vi "load_automatic.vi"(8 "error in (no error)":errorcluster) -> (0 "error out":errorcluster, 2 "replaced_step(s)":bool, 3 "automatic_steps out":variant)   [LabVIEW 2015, in "example_01.lvlib"]
doc: "load_automatic.vi will add automatic steps as variant attributes to an empty variant."
uses:
  example_01.lvlib
  <userlib>/antonio-alexander/lv-recipe-machine/public/_controls/step.ctl
  <userlib>/antonio-alexander/lv-recipe-machine/public/_controls/vi_reference_type.ctl
  _controls/steps_actions.ctl
  <userlib>/antonio-alexander/lv-recipe-machine/public/_controls/vi_reference_automatic_step.ctl
  <userlib>/antonio-alexander/lv-recipe-machine/public/_controls/vi_reference_criteria.ctl
  <userlib>/antonio-alexander/lv-recipe-machine/public/_controls/vi_reference_launch.ctl
  <userlib>/antonio-alexander/lv-recipe-machine/public/_controls/vi_reference_manual_action.ctl
  <userlib>/antonio-alexander/lv-recipe-machine/public/_controls/vi_reference_transition.ctl
  <userlib>/antonio-alexander/lv-recipe-machine/lv-recipe-machine.lvlib
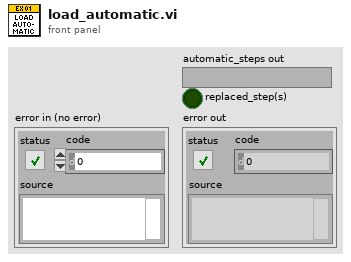
[diagram p1: front panel]
types:
  T1 = typedef "lv-recipe-machine.lvlib/vi_reference_type.ctl" = enum16{"<vi_reference_type>", "manual_action", "auto_step", "auto_criteria", "auto_transition", "auto_launcher", "<null>"}
  T2 = typedef "lv-recipe-machine.lvlib/vi_reference_transition.ctl" = refnum<vi>
  T3 = typedef "lv-recipe-machine.lvlib/vi_reference_manual_action.ctl" = refnum<vi>
  T4 = typedef "lv-recipe-machine.lvlib/vi_reference_launch.ctl" = refnum<vi>
  T5 = typedef "lv-recipe-machine.lvlib/vi_reference_criteria.ctl" = refnum<vi>
  T6 = typedef "lv-recipe-machine.lvlib/vi_reference_automatic_step.ctl" = refnum<vi>
  T7 = typedef "example_01.lvlib/steps_actions.ctl" = enum16{"<steps_actions>", "manual_random", "manual_comparison", "manual_wait", "auto_random", "auto_wait", "criteria_initialize", "criteria_count", "criteria_comparison", "transition_simple", "transition_count", "transition_comparison", "launch_wait", "<null>"}
  T8 = typedef "lv-recipe-machine.lvlib/step.ctl" = cluster{"name":string, "vi_reference":variant}
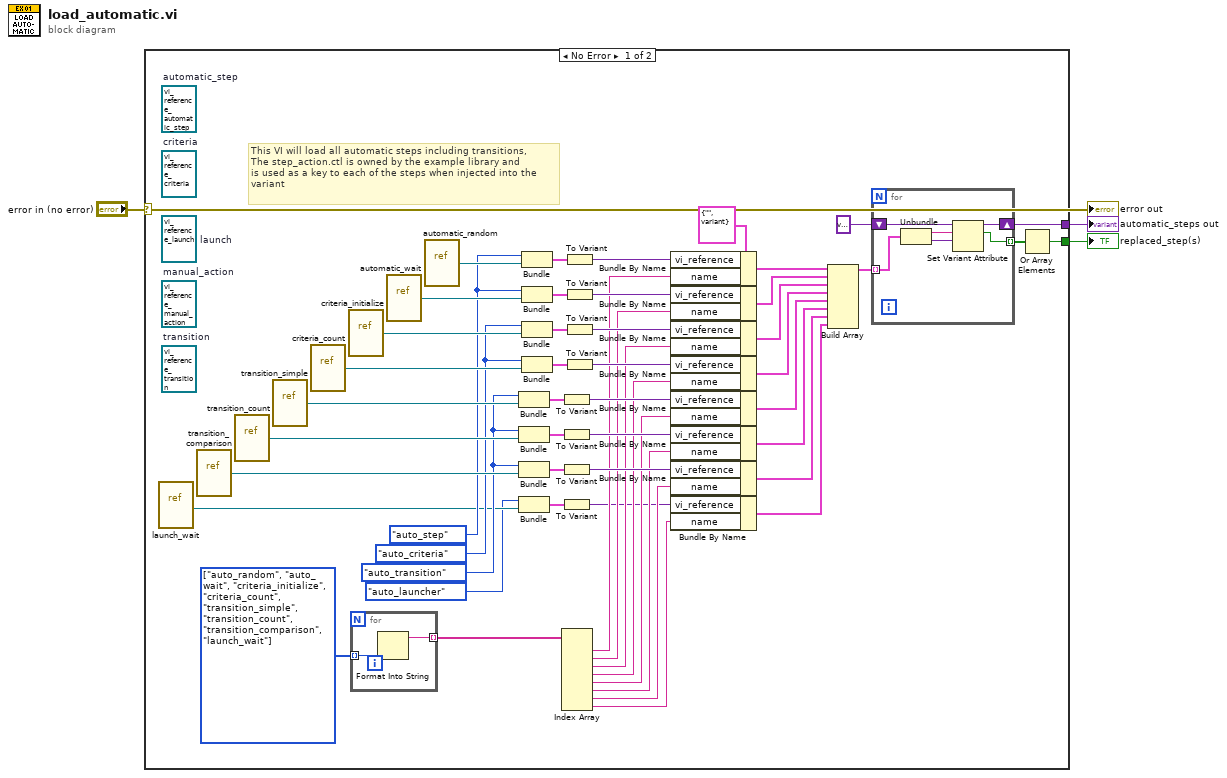
[diagram p0: block diagram]
diagram:
  n1 = case shown="No Error" "error in (no error)" {
    tunnel: [w54 _] -> w3
    tunnel: [w51 _] -> w2
    frame No Error {
      (unwired) T2 refnum  # transition
      (unwired) T3 refnum  # manual_action
      (unwired) T4 refnum  # launch
      (unwired) T5 refnum  # criteria
      (unwired) T6 refnum  # automatic_step
      w25 = T7[] [enum."auto_random", enum."auto_wait", enum."criteria_initialize", enum."criteria_count", enum."transition_simple", enum."transition_count", enum."transition_comparison", enum."launch_wait"] items=["<steps_actions>", "manual_random", "manual_comparison", "manual_wait", "auto_random", "auto_wait", "criteria_initialize", "criteria_count", "criteria_comparison", "transition_simple", "transition_count", "transition_comparison", "launch_wait", "<null>"]
      w28 = vi_reference_type."auto_transition" ("vi_reference_type")
      w27 = vi_reference_type."auto_criteria" ("vi_reference_type")
      w29 = vi_reference_type."auto_step" ("vi_reference_type")
      w10 = T8 {"name"="", "vi_reference"=variant(refnum<vi> refnum)} ("step")
      # "This VI will load all automatic steps including transitions, \nThe step_action.ctl is owned by the example library and\nis used as a key to each of the steps when injected into the\nvariant"
      n2 = vi-ref "launch_wait.vi"() -> (w5:refnum<vi>)
      n3 = vi-ref "transition_comparison.vi"() -> (w30:refnum<vi>)
      n4 = vi-ref "transition_count.vi"() -> (w31:refnum<vi>)
      n5 = vi-ref "transition_simple.vi"() -> (w55:refnum<vi>)
      n6 = vi-ref "criteria_count.vi"() -> (w47:refnum<vi>)
      n7 = vi-ref "criteria_initialize.vi"() -> (w36:refnum<vi>)
      n8 = for {
        tunnel: w25 -> [w57] mode=indexing
        tunnel: [w56] -> w24 mode=indexing
        n9 = Format Into String(w57) -> (resulting string=w56:string)  [unwired: 3 in, 1 out]
      }
      n10 = vi-ref "automatic_wait.vi"() -> (w48:refnum<vi>)
      n11 = vi-ref "automatic_random.vi"() -> (w49:refnum<vi>)
      n12 = Bundle("vi_reference_type"=w28, w55) -> (w38:cluster{"vi_reference_type":T1, refnum<vi>})  [unwired: 1 in]
      n13 = Bundle("vi_reference_type"=w28, w31) -> (w35:cluster{"vi_reference_type":T1, refnum<vi>})  [unwired: 1 in]
      n14 = Bundle("vi_reference_type"=w28, w30) -> (w34:cluster{"vi_reference_type":T1, refnum<vi>})  [unwired: 1 in]
      n15 = Bundle("vi_reference_type"=vi_reference_type."auto_launcher", w5) -> (w8:cluster{"vi_reference_type":T1, refnum<vi>})  [unwired: 1 in]
      n16 = Bundle("vi_reference_type"=w29, w49) -> (w41:cluster{"vi_reference_type":T1, refnum<vi>})  [unwired: 1 in]
      n17 = Bundle("vi_reference_type"=w29, w48) -> (w40:cluster{"vi_reference_type":T1, refnum<vi>})  [unwired: 1 in]
      n18 = Bundle("vi_reference_type"=w27, w36) -> (w42:cluster{"vi_reference_type":T1, refnum<vi>})  [unwired: 1 in]
      n19 = Bundle("vi_reference_type"=w27, w47) -> (w39:cluster{"vi_reference_type":T1, refnum<vi>})  [unwired: 1 in]
      n20 = To Variant(anything=w38) -> (Variant=w37:variant)
      n21 = To Variant(anything=w35) -> (Variant=w33:variant)
      n22 = To Variant(anything=w34) -> (Variant=w32:variant)
      n23 = To Variant(anything=w8) -> (Variant=w7:variant)
      n24 = Index Array(array=w24) -> (element #1=w23:string, element #2=w22:string, element #3=w21:string, element #4=w20:string, element #5=w19:string, element #6=w18:string, element #7=w17:string, element #8=w6:string)  [unwired: 8 in]
      n25 = To Variant(anything=w41) -> (Variant=w45:variant)
      n26 = To Variant(anything=w40) -> (Variant=w44:variant)
      n27 = To Variant(anything=w42) -> (Variant=w46:variant)
      n28 = To Variant(anything=w39) -> (Variant=w43:variant)
      n29 = Bundle By Name(cluster=w10, "vi_reference"=w45, "name"=w23) -> (w26:T8)
      n30 = Bundle By Name(cluster=w10, "vi_reference"=w44, "name"=w22) -> (w16:T8)
      n31 = Bundle By Name(cluster=w10, "vi_reference"=w46, "name"=w21) -> (w15:T8)
      n32 = Bundle By Name(cluster=w10, "vi_reference"=w43, "name"=w20) -> (w14:T8)
      n33 = Bundle By Name(cluster=w10, "vi_reference"=w37, "name"=w19) -> (w13:T8)
      n34 = Bundle By Name(cluster=w10, "vi_reference"=w33, "name"=w18) -> (w12:T8)
      n35 = Bundle By Name(cluster=w10, "vi_reference"=w32, "name"=w17) -> (w11:T8)
      n36 = Bundle By Name(cluster=w10, "vi_reference"=w7, "name"=w6) -> (w9:T8)
      n37 = Build Array(w26, w16, w15, w14, w13, w12, w11, w9) -> (w53:T8[])
      n38 = for {
        tunnel: w53 -> [w61] mode=indexing
        shift-right: [w62] -> w54
        shift-left: variant ("automatic_steps in") -> [w63]
        tunnel: [w59] -> w50 mode=indexing
        n39 = Unbundle(w61) -> ("name"=w60:string, "vi_reference"=w58:variant)
        n40 = Set Variant Attribute(Variant=w63, name=w60, value=w58) -> (Variant out=w62:variant, replaced=w59:bool)  [unwired: 1 in, 1 out]
      }
      n41 = Or Array Elements(Boolean array=w50) -> (logical OR=w51:bool)
    }
    frame Error {
    }
  }
  "automatic_steps out" <- w3
  "replaced_step(s)" <- w2
  "error out" <- "error in (no error)"
